vi "GOOP_Library_Item_Init.vi"(11 "Object":u64) -> ()   [LabVIEW 2020]
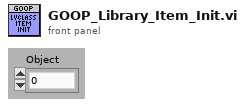
[diagram p1: front panel]
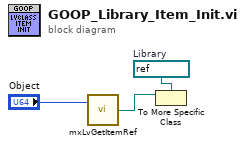
[diagram p0: block diagram]
diagram:
  w2 = refnum<vi> refnum  # Library
  n1 = call <resource>:"mxLvGetItemRef.vi"("Item"="Object") -> ("Item Refnum"=w1:refnum<vi>)  [unwired: 1 in, 2 out]
  n2 = To More Specific Class(target class=w2, reference=w1) -> ()  [unwired: 1 in, 2 out]
